vi "Emballage_BDD_GVF_result_update+chemin.vi"(8 "Error in":errorcluster caption="Error in (no error)", 10 "Tab codif-code bar IN":string[][](array[string]), 11 "Énum":enum16{"get", "set"}(ring)) -> (0 "Error out":errorcluster, 3 "Tab codif-code bar OUT":string[][](array[string]))   [LabVIEW 2020]
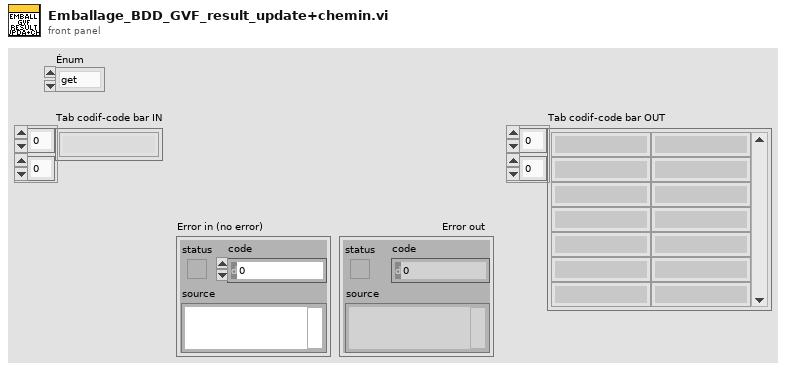
[diagram p1: front panel]
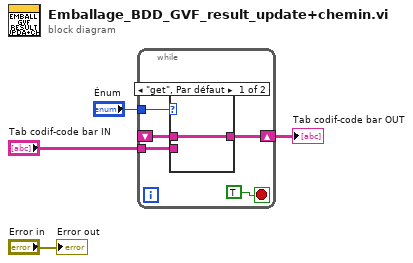
[diagram p0: block diagram]
diagram:
  n1 = while {
    tunnel: "Énum" -> [w8]
    tunnel: "Tab codif-code bar IN" -> [w5]
    shift-right: [w7] -> w3
    shift-left: _ -> [w6]
    stop <- TRUE stop-if-true
    n2 = case shown="\"get\", Par défaut" w8 {
      tunnel: [w10 w11] -> w7
      tunnel: w6 -> [w10 _]
      tunnel: w5 -> [_ w11]
      frame "get", Default {
      }
      frame "set" {
      }
    }
  }
  "Tab codif-code bar OUT" <- w3
  "Error out" <- "Error in"
